vi "uView_fp.get.vi"(8 "error in (no error)":errorcluster, 11 "uView in":refnum<class "uView.lvclass">) -> (0 "error out":errorcluster, 2 "VI Refnum":refnum<vi>, 3 "uView out":refnum<class "uView.lvclass">)   [LabVIEW 2023, in "uLib.lvlib" / "uView.lvclass"]
doc: "Protected accessor method to GET the VI refnum of the FP."
uses:
  uView.lvclass
  uView.lvclass/uView.ctl
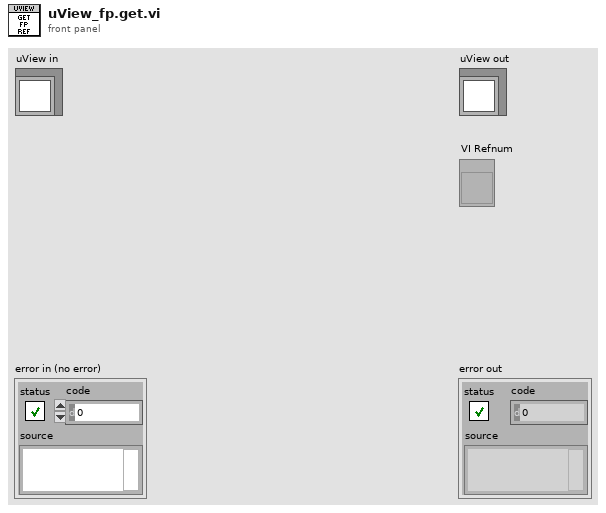
[diagram p1: front panel]
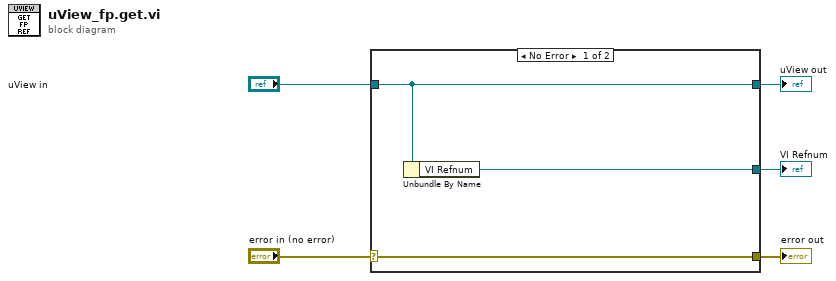
[diagram p0: block diagram]
diagram:
  n1 = case shown="No Error" "error in (no error)" {
    selector: "error in (no error)" -> [w8 w9]
    tunnel: [w8 w9] -> w4
    tunnel: [w7 w10] -> w2
    tunnel: "uView in" -> [w7 w10]
    tunnel: [w6 _] -> w1
    frame No Error {
      n2 = Unbundle By Name(w7) -> ("VI Refnum"=w6:refnum<vi>)
    }
    frame Error {
    }
  }
  "error out" <- w4
  "uView out" <- w2
  "VI Refnum" <- w1
